vi "Check_Status.vi"(2 "error in":errorcluster, 3 "instrument handle in":refnum<k15>) -> (0 "error out":errorcluster, 1 "instrument handle out":refnum<k15>)   [LabVIEW 2011]
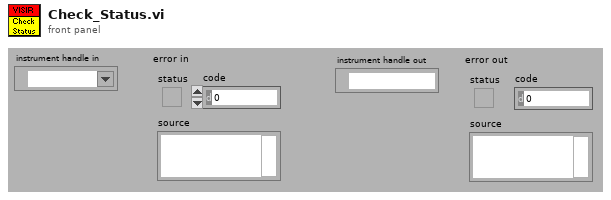
[diagram p1: front panel]
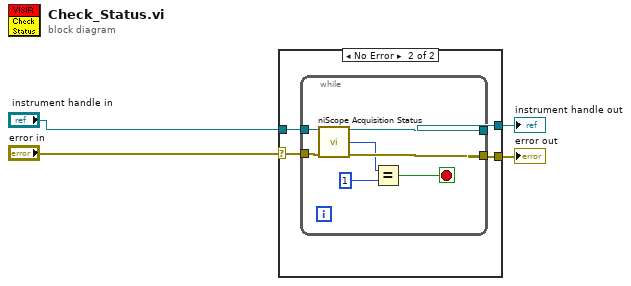
[diagram p0: block diagram]
diagram:
  n1 = case shown="No Error" "error in" {
    selector: "error in" -> [w6 w7]
    tunnel: [w6 w10] -> w4
    tunnel: [w5 w9] -> w3
    tunnel: "instrument handle in" -> [w5 w8]
    frame Error {
    }
    frame No Error {
      n2 = while {
        tunnel: w8 -> [w12]
        tunnel: [w17] -> w9
        tunnel: [w16] -> w10
        tunnel: w7 -> [w11]
        stop <- w13 stop-if-true
        n3 = call <instrlib>:"niScope Acquisition Status.vi"("instrument handle"=w12, "error in"=w11) -> ("instrument handle out"=w17:refnum<k15>, "acquisition status"=w15:i32, "error out"=w16:errorcluster)  [unwired: 11 in]
        n4 = Equal?(x=w15, y=1) -> (x = y?=w13:bool)
      }
    }
  }
  "error out" <- w4
  "instrument handle out" <- w3
